vi "SensorsToString.vi"(8 "error in (no error)":errorcluster, 11 "Sensors":T1) -> (0 "error out":errorcluster, 3 "Sensors String":string)   [LabVIEW 2012]
uses:
  2013-Competition_Dash/SensorsOutput.ctl
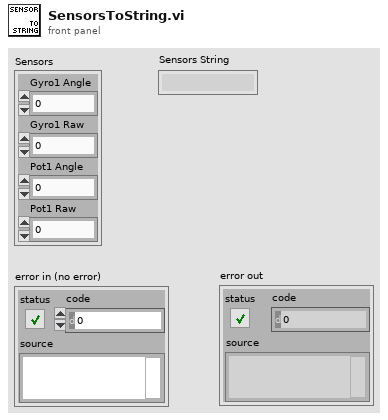
[diagram p1: front panel]
types:
  T1 = typedef "SensorsOutput.ctl" = cluster{"Gyro1 Angle":dbl, "Gyro1 Raw":dbl, "Pot1 Angle":dbl, "Pot1 Raw":dbl}
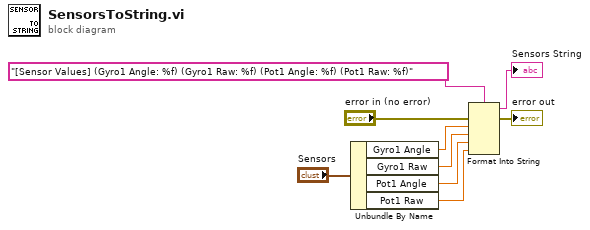
[diagram p0: block diagram]
diagram:
  n1 = Unbundle By Name("Sensors") -> ("Gyro1 Angle"=w6:dbl, "Gyro1 Raw"=w5:dbl, "Pot1 Angle"=w4:dbl, "Pot1 Raw"=w3:dbl)
  n2 = Format Into String(format string="[Sensor Values] (Gyro1 Angle: %f) (Gyro1 Raw: %f) (Pot1 Angle: %f) (Pot1 Raw: %f)", error in="error in (no error)", w6, w5, w4, w3) -> (resulting string=→"Sensors String":string, error out=→"error out":errorcluster)  [unwired: 1 in]
